vi "replace bad readings.vi"(8 "Meter reading in":sgl, 10 "bad data read":bool, 11 "Unit ID":i32) -> (0 "Meter reading out":dbl)   [LabVIEW 2019]
panel:
  out "Previous data":T1(array[cluster])
  out "all bad":bool
  out "x-1":i32
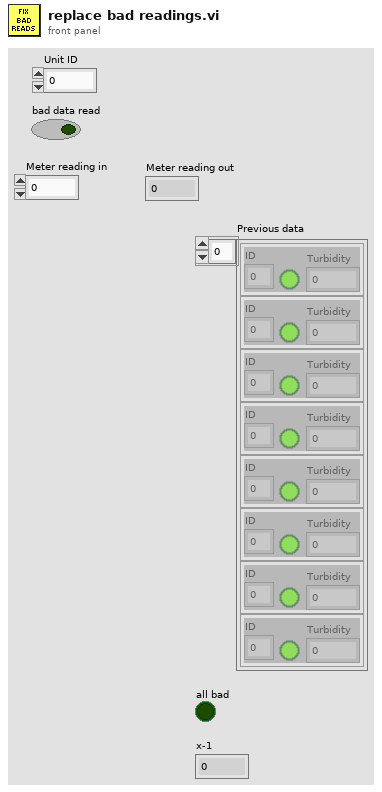
[diagram p1: front panel]
types:
  T1 = cluster{"ID":dbl, "Failed":bool, "Turbidity":dbl}[]
  T2 = cluster{"ID":dbl, "Failed":bool, "Turbidity":dbl}
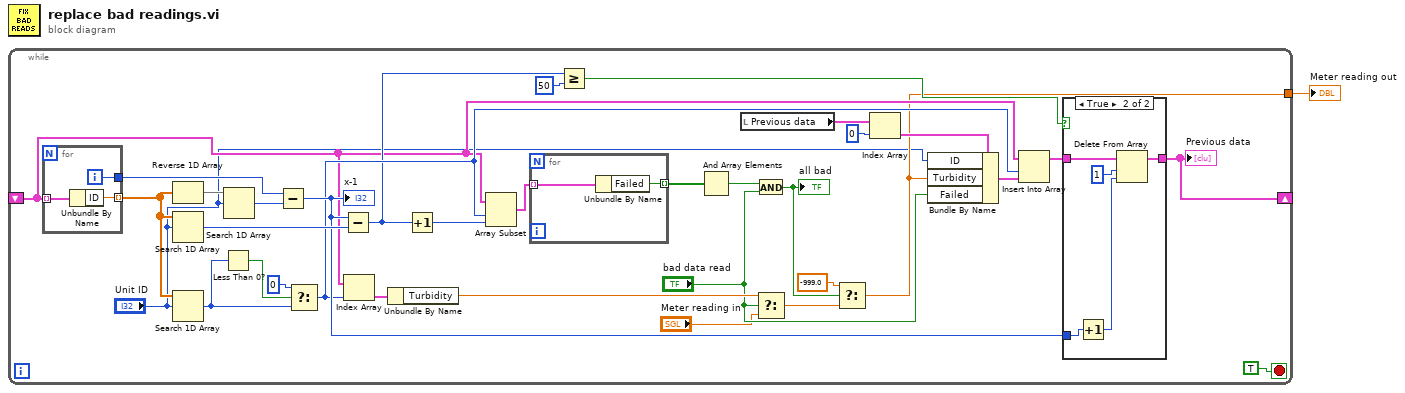
[diagram p0: block diagram]
diagram:
  n1 = while {
    tunnel: [w7] -> w1
    shift-right: [w6] -> _
    shift-left: _ -> [w8]
    stop <- TRUE stop-if-true
    n2 = for {
      tunnel: w8 -> [w40] mode=indexing
      tunnel: [w39] -> w15 mode=indexing
      tunnel: [w38] -> w14
      i -> [w38]
      n3 = Unbundle By Name(w40) -> ("ID"=w39:dbl)
    }
    n4 = Reverse 1D Array(array=w15) -> (reversed array=w31:dbl[])
    n5 = Search 1D Array(1D array=w15, element="Unit ID") -> (index of element=w27:i32)  [unwired: 1 in]
    n6 = Search 1D Array(1D array=w15, element="Unit ID") -> (index of element=w25:i32)  [unwired: 1 in]
    n7 = Less Than 0?(x=w25) -> (x < 0?=w26:bool)
    n8 = Search 1D Array(1D array=w31, element="Unit ID") -> (index of element=w30:i32)  [unwired: 1 in]
    n9 = Subtract(x=w14, y=w30) -> (x-y=w21:i32)
    "x-1" <- w21
    n10 = Select(t=0 ("index of element"), s=w26, f=w25) -> (s? t:f=w19:i32)
    n11 = Subtract(x=w21, y=w27) -> (x-y=w18:i32)
    n12 = Index Array(array=w8, index=w19) -> (element=w23:T2)
    n13 = Unbundle By Name(w23) -> ("Turbidity"=w22:dbl)
    n14 = Increment(x=w18) -> (x+1=w17:i32)
    n15 = Array Subset(array=w8, index=w19, length=w17) -> (w16:T1)
    n16 = for {
      tunnel: w16 -> [w37] mode=indexing
      tunnel: [w36] -> w13 mode=indexing
      n17 = Unbundle By Name(w37) -> ("Failed"=w36:bool)
    }
    n18 = Greater Or Equal?(x=w18, y=50) -> (x >= y?=w28:bool)
    n19 = And Array Elements(Boolean array=w13) -> (logical AND=w10:bool)
    n20 = local read "Previous data"() -> (w5:T1)
    n21 = And(x=w10, y="bad data read") -> (x .and. y?=w9:bool)
    "all bad" <- w9
    n22 = Select(t=w22, s="bad data read", f="Meter reading in") -> (s? t:f=w11:dbl)
    n23 = Select(t=-999.0, s=w9, f=w11) -> (s? t:f=w7:dbl)
    n24 = Index Array(array=w5, index=0) -> (element=w33:T2)
    n25 = Bundle By Name(cluster=w33, "ID"="Unit ID", "Turbidity"=w7, "Failed"="bad data read") -> (w32:T2)
    n26 = Insert Into Array(array=w8, index=w19, new element=w32) -> (w20:T1)
    n27 = case shown="True" w28 {
      tunnel: w20 -> [w41 w46]
      tunnel: [w41 w45] -> w6
      tunnel: w21 -> [_ w44]
      frame False {
      }
      frame True {
        n28 = Increment(x=w44) -> (x+1=w42:i32)
        n29 = Delete From Array(array=w46, length=1, index=w42) -> (array with subset deleted=w45:T1)  [unwired: 1 out]
      }
    }
    "Previous data" <- w6
  }
  "Meter reading out" <- w1
